vi "IOControl.vi"() -> ()   [LabVIEW 2011]
uses:
  API/API DYM.lvlib
panel:
  out "solenstatue output":i32[](array[numeric])
  in  "获取继电器状态按钮":bool
  in  "platformstatue":i32
  in  "platformNum":i32
  in  "solenstatue":i32
  in  "solenNum":i32
  in  "平台继电器动作按钮":bool
  in  "单个继电器动作按钮":bool
  out "布尔":bool
  in  "启动按钮":bool
  in  "退出按钮":bool
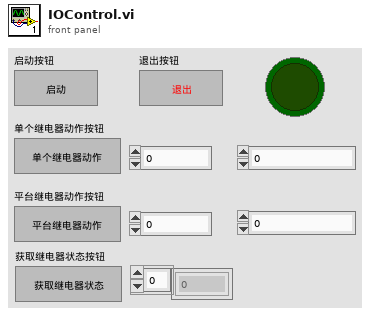
[diagram p1: front panel]
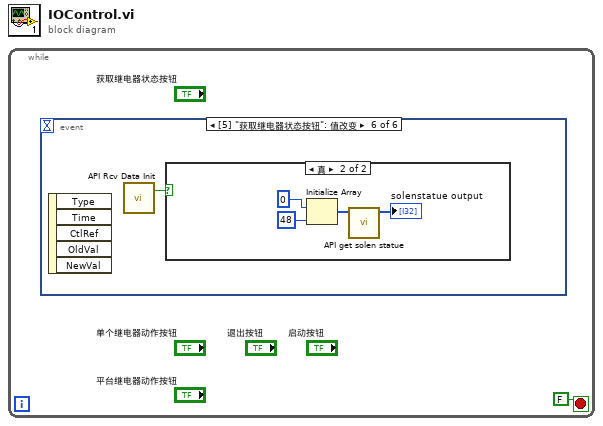
[diagram p0: block diagram]
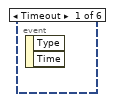
[diagram p2: hidden frame]
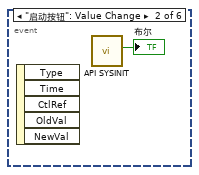
[diagram p3: hidden frame]
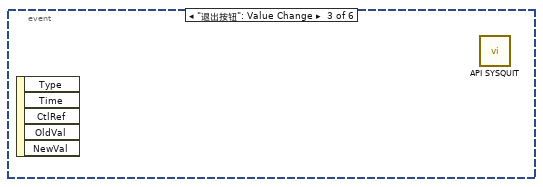
[diagram p4: hidden frame]
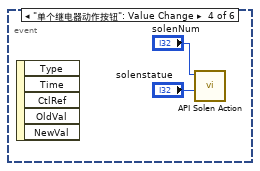
[diagram p5: hidden frame]
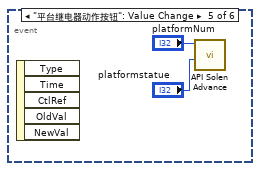
[diagram p6: hidden frame]
diagram:
  n1 = while {
    stop <- FALSE stop-if-true
    n2 = event shown="[5] \"获取继电器状态按钮\": 值改变" {
      selector: _ -> [_ _ _ _ _ _]
      dyn-events: _ -> [_ _ _ _ _ _]
      timeout: _ -> [_ _ _ _ _ _]
      event Timeout {
        n3 = event-data() -> ()  [unwired: 1 in, 2 out]
      }
      event "启动按钮": Value Change {
        n4 = event-data() -> ()  [unwired: 1 in, 5 out]
        n5 = call "API SYSINIT.vi"() -> ("SYSINIT return value"=→"布尔":bool)  [unwired: 11 in]
      }
      event "退出按钮": Value Change {
        n6 = event-data() -> ()  [unwired: 1 in, 5 out]
        n7 = call "API SYSQUIT.vi"() -> ()  [unwired: 12 in]
      }
      event "单个继电器动作按钮": Value Change {
        n8 = event-data() -> ()  [unwired: 1 in, 5 out]
        n9 = call "API Solen Action.vi"("statue"="solenstatue", "solenNum"="solenNum") -> ()  [unwired: 9 in, 1 out]
      }
      event "平台继电器动作按钮": Value Change {
        n10 = event-data() -> ()  [unwired: 1 in, 5 out]
        n11 = call "API Solen Advance.vi"("statue"="platformstatue", "platformNum"="platformNum") -> ()  [unwired: 9 in, 1 out]
      }
      event "获取继电器状态按钮": Value Change {
        n12 = event-data() -> ()  [unwired: 1 in, 5 out]
        n13 = call "API Rcv Data Init.vi"() -> ("RTV"=w7:bool)  [unwired: 2 in, 1 out]
        n14 = case shown="真" w7 {
          frame False {
          }
          frame True {
            n15 = Initialize Array(0 ("元素"), 48 ("维数大小")) -> (w9:i32[])
            n16 = call "API get solen statue.vi"("solenstatue input"=w9) -> ("solenstatue output"=→"solenstatue output":i32[])  [unwired: 10 in]
          }
        }
      }
    }
  }
